vi "Abre pasta.vi"(0 "Pasta do ensaio":path) -> (1 "Dados":string, 2 "Infos para processamento out":T1={"Diâmetro do furo [mm]"=1.4, "Diâmetro da linha média [mm]"=5.0, "IncF"=0.2, "Módulo de elasticidade [GPa]"=207.0, "Módulo de Poisson"=0.3, "Tipo de roseta utilizada"=enum."Tipo A", "Método de análise"=enum."Simplificado 2008", "Pfinal"=0.3, "Parar auto."=TRUE})   [LabVIEW 2016]
uses:
  Controles/Infos para processamento.ctl
panel:
  in  "Confirmar dados":bool
  in  "Infos para processamento":T1={"Diâmetro do furo [mm]"=1.4, "Diâmetro da linha média [mm]"=5.0, "IncF"=0.2, "Módulo de elasticidade [GPa]"=207.0, "Módulo de Poisson"=0.3, "Tipo de roseta utilizada"=enum."Tipo A", "Método de análise"=enum."Simplificado 2008", "Pfinal"=0.3, "Parar auto."=TRUE}
  # "Estes foram os dados encontrados no arquivo de informações. Eles estão corretos?"
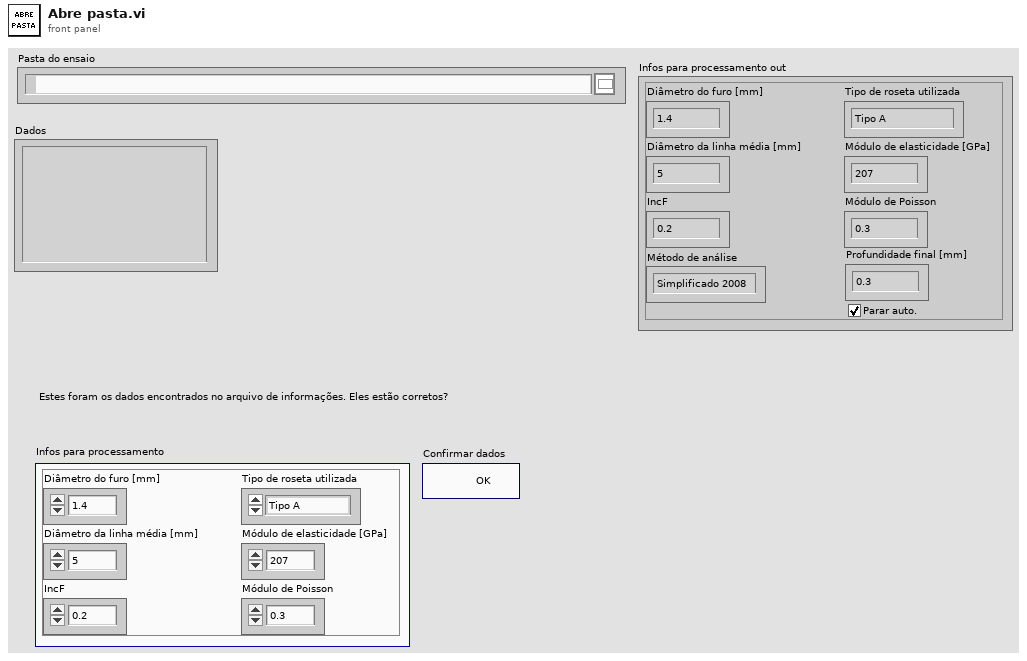
[diagram p1: front panel]
types:
  T1 = typedef "Infos para processamento.ctl" = cluster{"Diâmetro do furo [mm]":dbl, "Diâmetro da linha média [mm]":dbl, "IncF":dbl, "Módulo de elasticidade [GPa]":dbl, "Módulo de Poisson":dbl, "Tipo de roseta utilizada":enum16{"Tipo A", "Tipo B", "Tipo C"}, "Método de análise":enum16{"Não uniforme 2013", "Simplificado 2013", "Simplificado 2008"}, "Pfinal":dbl, "Parar auto.":bool}
  T2 = enum16{"Não uniforme 2013", "Simplificado 2013", "Simplificado 2008"}
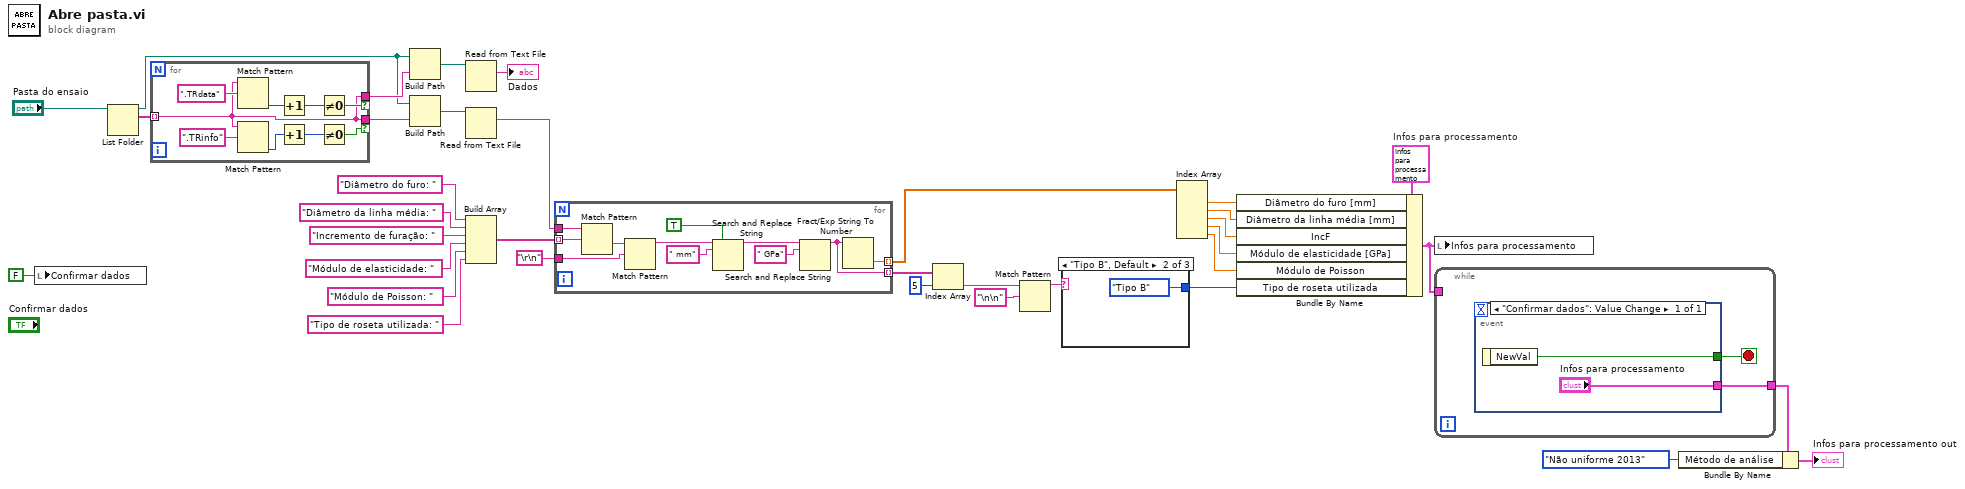
[diagram p0: block diagram]
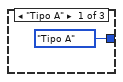
[diagram p2: hidden frame]
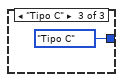
[diagram p3: hidden frame]
diagram:
  w18 = T1 {"Diâmetro do furo [mm]"=1.4, "Diâmetro da linha média [mm]"=5.0, "IncF"=0.2, "Módulo de elasticidade [GPa]"=207.0, "Módulo de Poisson"=0.3, "Tipo de roseta utilizada"=enum."Tipo A", "Método de análise"=enum."Simplificado 2008", "Pfinal"=0.3, "Parar auto."=TRUE}  # Infos para processamento
  n1 = local write "Confirmar dados"(FALSE ("Confirmar dados")) -> ()
  n2 = List Folder(path="Pasta do ensaio") -> (path out=w30:path, filenames=w34:string[])  [unwired: 3 in, 2 out]
  n3 = for {
    tunnel: w34 -> [w36] mode=indexing
    tunnel: [w36] -> w33 if=w40
    tunnel: [w36] -> w29 if=w37
    n4 = Match Pattern(string=w36, regular expression=".TRdata") -> (offset past match=w42:i32)  [unwired: 1 in, 3 out]
    n5 = Match Pattern(string=w36, regular expression=".TRinfo") -> (offset past match=w38:i32)  [unwired: 1 in, 3 out]
    n6 = Increment(x=w42) -> (x+1=w41:i32)
    n7 = Increment(x=w38) -> (x+1=w39:i32)
    n8 = Not Equal To 0?(x=w41) -> (x != 0?=w40:bool)
    n9 = Not Equal To 0?(x=w39) -> (x != 0?=w37:bool)
  }
  n10 = Build Path(base path=w30, name or relative path=w33) -> (appended path=w32:path)
  n11 = Build Path(base path=w30, name or relative path=w29) -> (appended path=w31:path)
  n12 = Read from Text File(file (use dialog)=w32) -> (text=→"Dados":string)  [unwired: 3 in, 3 out]
  n13 = Read from Text File(file (use dialog)=w31) -> (text=w21:string)  [unwired: 3 in, 3 out]
  n14 = Build Array("Diâmetro do furo: " ("string"), "Diâmetro da linha média: " ("string"), "Incremento de furação: " ("string"), "Módulo de elasticidade: " ("string"), "Módulo de Poisson: " ("string"), "Tipo de roseta utilizada: " ("string")) -> (w20:string[])
  n15 = for {
    tunnel: w21 -> [w55]
    tunnel: w20 -> [w54] mode=indexing
    tunnel: "\r\n" -> [w52]
    tunnel: [w46] -> w17 mode=indexing
    tunnel: [w45] -> w16 mode=indexing
    n16 = Match Pattern(string=w55, regular expression=w54) -> (after substring=w53:string)  [unwired: 1 in, 3 out]
    n17 = Match Pattern(string=w53, regular expression=w52) -> (before substring=w51:string)  [unwired: 1 in, 3 out]
    n18 = Search and Replace String(replace all?=TRUE ("replace all? (F)"), input string=w51, search string=" mm") -> (result string=w47:string)  [unwired: 5 in, 3 out]
    n19 = Search and Replace String(input string=w47, search string=" GPa") -> (result string=w46:string)  [unwired: 6 in, 3 out]
    n20 = Fract/Exp String To Number(string=w46) -> (number=w45:dbl)  [unwired: 3 in, 1 out]
  }
  n21 = Index Array(array=w17, index=5) -> (element=w7:string)
  n22 = Match Pattern(string=w7, regular expression="\n\n") -> (before substring=w6:string)  [unwired: 1 in, 3 out]
  n23 = case shown="\"Tipo B\", Default" w6 {
    tunnel: [enum16{"Tipo A", "Tipo B", "Tipo C"}."Tipo A" ("Tipo de roseta utilizada") enum16{"Tipo A", "Tipo B", "Tipo C"}."Tipo B" ("Tipo de roseta utilizada") enum16{"Tipo A", "Tipo B", "Tipo C"}."Tipo C" ("Tipo de roseta utilizada")] -> w8
    frame "Tipo A" {
    }
    frame "Tipo B", Default {
    }
    frame "Tipo C" {
    }
  }
  n24 = Index Array(array=w16) -> (element #1=w15:dbl, element #2=w14:dbl, element #3=w13:dbl, element #4=w12:dbl, element #5=w11:dbl)  [unwired: 5 in]
  n25 = Bundle By Name(cluster=w18, "Diâmetro do furo [mm]"=w15, "Diâmetro da linha média [mm]"=w14, "IncF"=w13, "Módulo de elasticidade [GPa]"=w12, "Módulo de Poisson"=w11, "Tipo de roseta utilizada"=w8) -> (w10:T1)
  n26 = local write "Infos para processamento"(w10) -> ()
  n27 = while {
    tunnel: [w60] -> w3
    tunnel: w10 -> [_]
    stop <- w59 stop-if-true
    n28 = event shown="[0] \"Confirmar dados\": Value Change" {
      selector: _ -> [_]
      dyn-events: _ -> [_]
      timeout: _ -> [_]
      tunnel: ["Infos para processamento"] -> w60
      tunnel: [w61] -> w59
      event "Confirmar dados": Value Change {
        n29 = event-data() -> ("NewVal"=w61:bool)  [unwired: 1 in]
      }
    }
  }
  n30 = Bundle By Name(cluster=w3, "Método de análise"=T2."Não uniforme 2013") -> (→"Infos para processamento out":T1)
